vi "getState.vi"(8 "error in (no error)":errorcluster, 11 "MonoState in":refnum<class "MonoState.lvclass">) -> (0 "error out":errorcluster, 2 "DeviceStatus":T1, 3 "MonoState out":refnum<class "MonoState.lvclass">)   [LabVIEW 2016, in "MonoState.lvclass"]
uses:
  MonoState.lvclass
  Typedefs/DeviceStatus.ctl
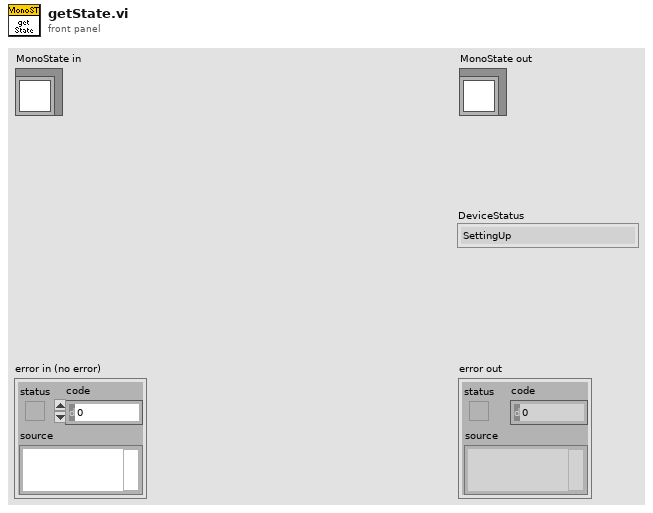
[diagram p1: front panel]
types:
  T1 = typedef "DeviceStatus.ctl" = enum16{"SettingUp", "Ready", "Offline", "Fault"}
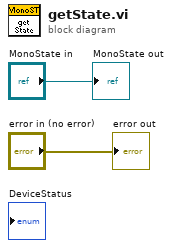
[diagram p0: block diagram]
diagram:
  "error out" <- "error in (no error)"
  "MonoState out" <- "MonoState in"
